vi "2일차10vi.vi"() -> ()   [LabVIEW 2014]
panel:
  out "강도 그래프 2":dbl[][](graph)
  out "강도 그래프":dbl[][](graph)
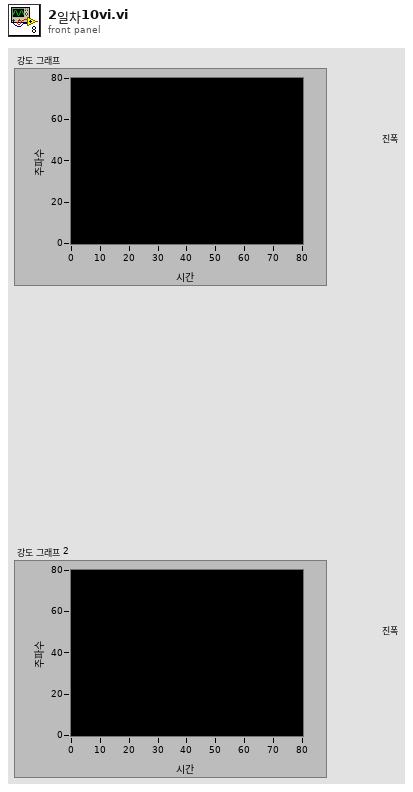
[diagram p1: front panel]
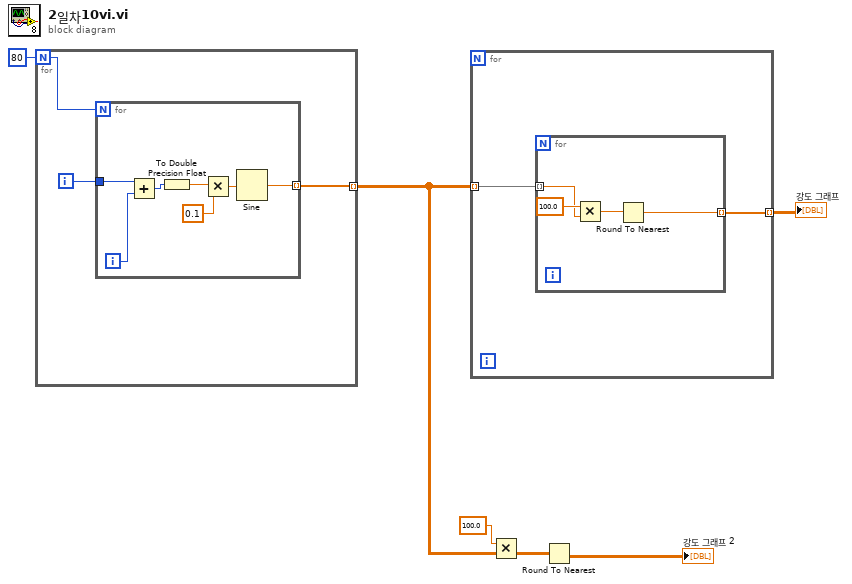
[diagram p0: block diagram]
diagram:
  n1 = for {
    N: 80 -> [w9]
    tunnel: [w7] -> w5 mode=indexing
    i -> [w8]
    n2 = for {
      N: w9 -> [_]
      tunnel: w8 -> [w16]
      tunnel: [w10] -> w7 mode=indexing
      i -> [w15]
      n3 = Add(x=w16, y=w15) -> (x+y=w14:i32)
      n4 = To Double Precision Float(number=w14) -> (double precision float=w13:dbl)
      n5 = Multiply(x=w13, y=0.1 ("x")) -> (x*y=w11:dbl)
      n6 = Sine(x=w11) -> (sin(x)=w10:dbl)
    }
  }
  n7 = for {
    tunnel: w5 -> [w18] mode=indexing
    tunnel: [w17] -> w4 mode=indexing
    n8 = for {
      tunnel: w18 -> [w20] mode=indexing
      tunnel: [w19] -> w17 mode=indexing
      n9 = Multiply(x=100.0, y=w20) -> (x*y=w21:dbl)
      n10 = Round To Nearest(number=w21) -> (nearest integer value=w19:dbl)
    }
  }
  "강도 그래프" <- w4
  n11 = Multiply(x=100.0, y=w5) -> (x*y=w3:dbl[][])
  n12 = Round To Nearest(number=w3) -> (nearest integer value=→"강도 그래프 2":dbl[][])
